vi "Configure TS Panel.vi"(8 "error in (no error)":errorcluster, 11 "Generic Test Stand in":refnum<class "Generic Test Stand.lvclass">) -> (0 "error out":errorcluster, 3 "Generic Test Stand out":refnum<class "Generic Test Stand.lvclass">)   [LabVIEW 2019, in "Generic Test Stand.lvclass"]
uses:
  Generic Test Stand.lvclass
  Generic Test Stand.lvclass/Generic Test Stand.ctl
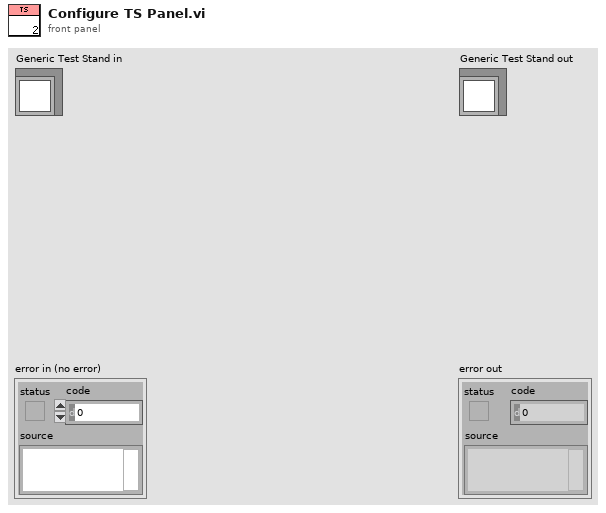
[diagram p1: front panel]
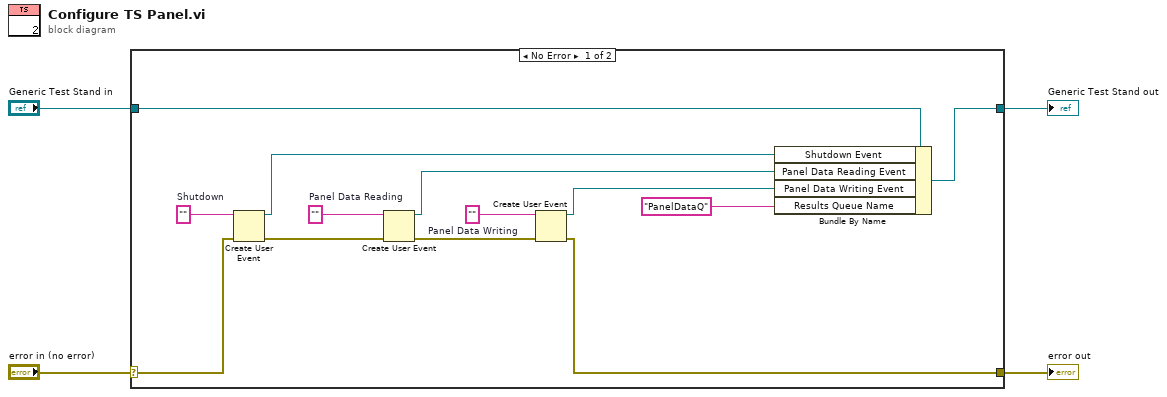
[diagram p0: block diagram]
diagram:
  n1 = case shown="No Error" "error in (no error)" {
    selector: "error in (no error)" -> [w10 w19]
    tunnel: [w6 w19] -> w3
    tunnel: [w5 w18] -> w1
    tunnel: "Generic Test Stand in" -> [w17 w18]
    frame No Error {
      w14 = ""  # Panel Data Writing
      w15 = ""  # Panel Data Reading
      w16 = ""  # Shutdown
      n2 = Create User Event(user event datatype=w16, error in=w10) -> (user event=w13:refnum<user-event>, error out=w9:errorcluster)
      n3 = Create User Event(user event datatype=w15, error in=w9) -> (user event=w12:refnum<user-event>, error out=w8:errorcluster)
      n4 = Create User Event(user event datatype=w14, error in=w8) -> (user event=w11:refnum<user-event>, error out=w6:errorcluster)
      n5 = Bundle By Name(cluster=w17, "Shutdown Event"=w13, "Panel Data Reading Event"=w12, "Panel Data Writing Event"=w11, "Results Queue Name"="PanelDataQ" ("name (unnamed)")) -> (w5:refnum<class "Generic Test Stand.lvclass">)
    }
    frame Error {
    }
  }
  "error out" <- w3
  "Generic Test Stand out" <- w1
